vi "svl_Equivalent Continuous Resampled Level with IC.vi"(6 "state in":cluster{dbl, dbl} {"?" format="%.2f"}, 8 "error in (no error)":errorcluster, 9 "processing state":T2(ring), 11 "even angle signal":T1 {"even angle signal" format="%.2f"; "dr" format="%.2f"; "r0" format="%.2f"}) -> (0 "error out":errorcluster, 3 "Numeric":dbl format="%.2f", 4 "state out":cluster{dbl, dbl} {"?" format="%.2f"})   [LabVIEW 2017]
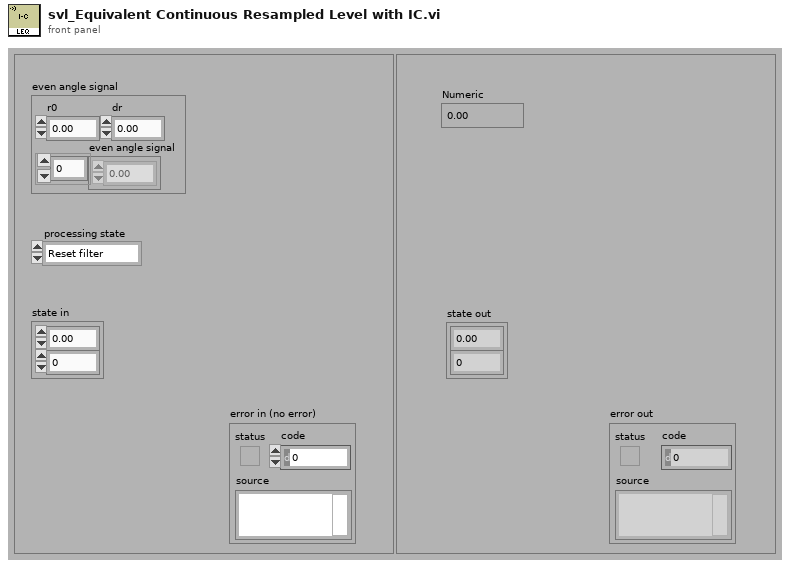
[diagram p1: front panel]
types:
  T1 = cluster{"r0":dbl, "dr":dbl, "even angle signal":dbl[]}
  T2 = enum16{"Reset filter", "Restart averaging", "Continue processing"}
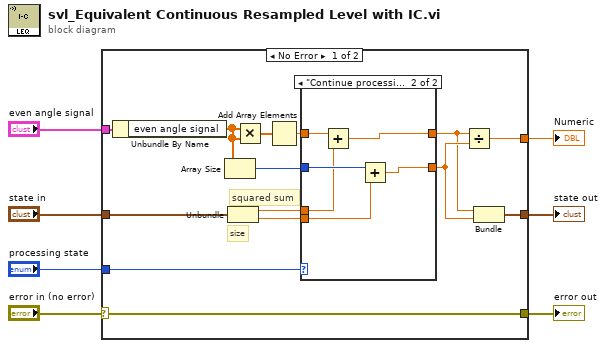
[diagram p0: block diagram]
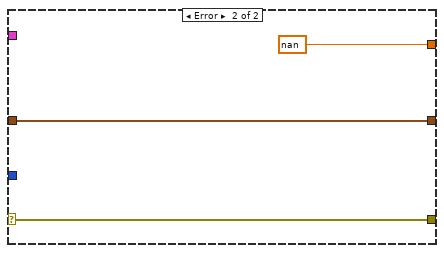
[diagram p3: hidden frame]
diagram:
  n1 = case shown="No Error" "error in (no error)" {
    selector: "error in (no error)" -> [w11 w32]
    tunnel: "state in" -> [w21 w31]
    tunnel: [w18 w31] -> w6
    tunnel: [w15 nan] -> w5
    tunnel: "processing state" -> [w14 _]
    tunnel: "even angle signal" -> [w9 _]
    tunnel: [w11 w32] -> w1
    frame No Error {
      # "squared sum"
      # "size"
      n2 = Unbundle By Name(w9) -> ("even angle signal"=w8:dbl[])
      n3 = Array Size(array=w8) -> (size(s)=w10:i32)
      n4 = Unbundle(w21) -> (w19:dbl, w20:dbl)
      n5 = Multiply(x=w8, y=w8) -> (x*y=w12:dbl[])
      n6 = Add Array Elements(numeric array=w12) -> (sum=w13:dbl)
      n7 = case shown="\"Continue processing\"" w14 {
        tunnel: w13 -> [w23 w26]
        tunnel: w10 -> [w22 w29]
        tunnel: [w22 w28] -> w17
        tunnel: [w23 w27] -> w16
        tunnel: w19 -> [_ w25]
        tunnel: w20 -> [_ w24]
        frame "Reset filter", "Restart averaging", Default {
        }
        frame "Continue processing" {
          n8 = Add(x=w26, y=w25) -> (x+y=w27:dbl)
          n9 = Add(x=w29, y=w24) -> (x+y=w28:dbl)
        }
      }
      n10 = Divide(x=w16, y=w17) -> (x/y=w15:dbl)
      n11 = Bundle(w16, w17) -> (w18:cluster{dbl, dbl})  [unwired: 1 in]
    }
    frame Error {
    }
  }
  "state out" <- w6
  "Numeric" <- w5
  "error out" <- w1
